vi "_testRTseqBug.vi"(11 "Sequence Context In":refnum<k7>) -> (0 "error out":errorcluster, 3 "Report Text":string)   [LabVIEW 2020]
panel:
  in  "type":enum16{"bool", "number"}(ring)
  in  "stop":bool
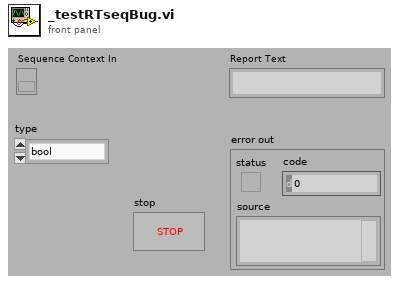
[diagram p1: front panel]
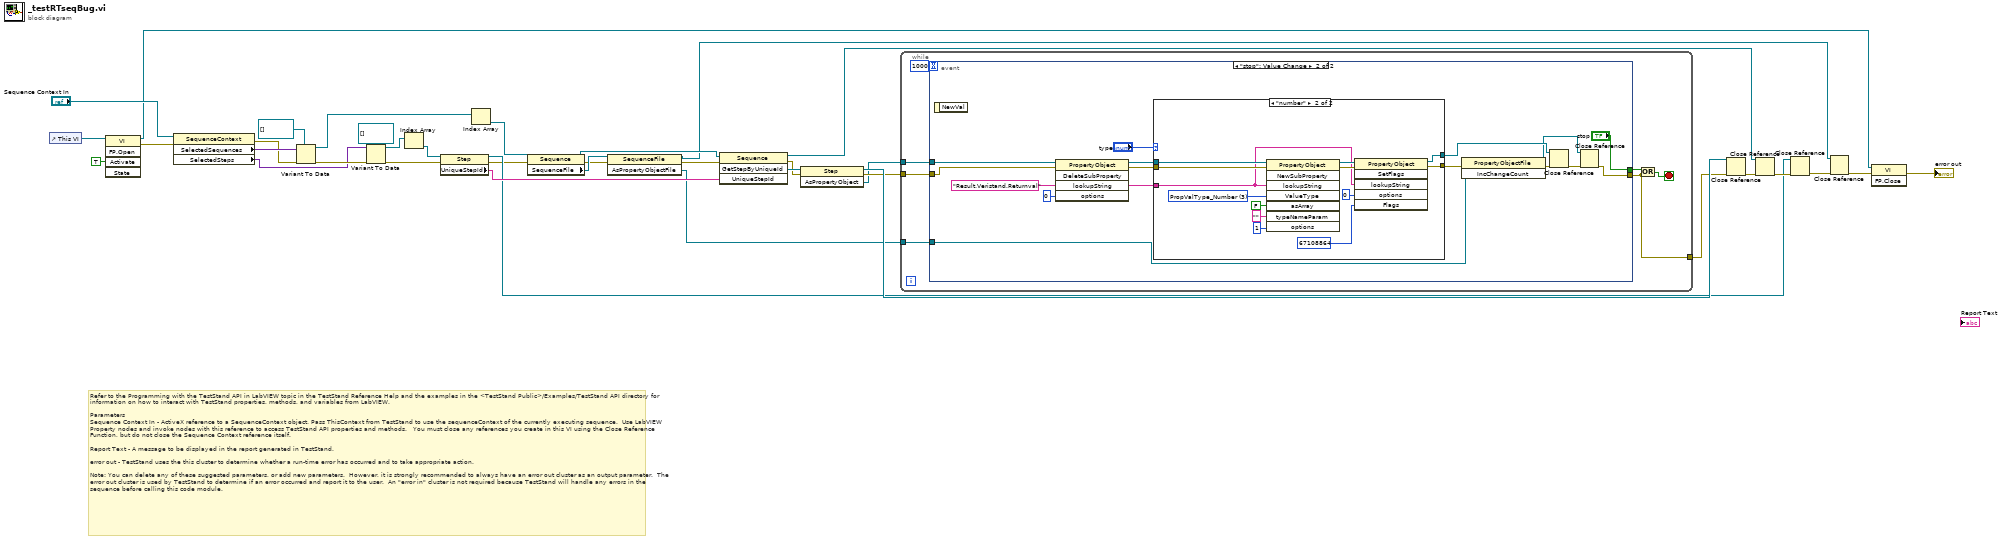
[diagram p0: block diagram]
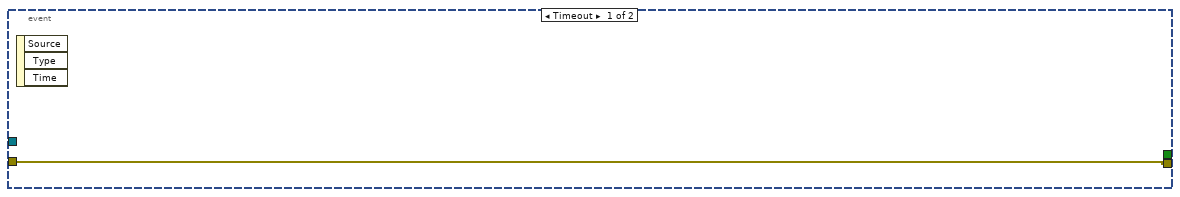
[diagram p2: hidden frame]
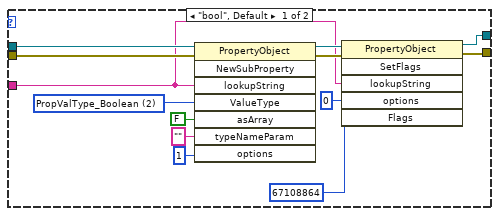
[diagram p3: hidden frame]
diagram:
  # "Refer to the Programming with the TestStand API in LabVIEW topic in the TestStand Reference Help and the examples in the <TestStand Public>/Examples/TestStand API directory for information on how to interact with TestStand properties, methods, and variables from LabVIEW.\n\nParameters\nSequence Context In - ActiveX reference to a SequenceContext object. Pass ThisContext from TestStand to use the sequenceContext of the currently executing sequence.  Use LabVIEW Property nodes and invoke nodes with this reference to access TestStand API properties and methods.   You must close any references you create in this VI using the Close Reference Function, but do not close the Sequence Context reference itself.\n\nReport Text - A message to be displayed in the report generated in TestStand. \n\nerror out - TestStand uses the this cluster to determine whether a run-time error has occurred and to take appropriate action.  \n\nNote: You can delete any of these suggested parameters, or add new parameters.  However, it is strongly recommended to always have an error out cluster as an output parameter.  The error out cluster is used by TestStand to determine if an error occurred and report it to the user.  An \"error in\" cluster is not required because TestStand will handle any errors in the sequence before calling this code module."
  n1 = control-ref of="This VI"() -> (w3:refnum<vi>)
  n2 = invoke class="VI" method="FP.Open"(reference=w3, "Activate"=TRUE ("Activate?")) -> (reference out=w2:refnum<vi>, error out=w4:errorcluster)  [unwired: 3 in, 3 out]
  n3 = property class="SequenceContext"(reference="Sequence Context In", error in=w4) -> (error out=w35:errorcluster, "SelectedSequences"=w36:variant, "SelectedSteps"=w31:variant)  [unwired: 1 out]
  n4 = Variant To Data(error in=w35, type=refnum<k7>[] [] ("Sequence"), Variant=w36) -> (data=w33:refnum<k7>[], error out=w32:errorcluster)
  n5 = Variant To Data(error in=w32, type=refnum<k7>[] [] ("Step"), Variant=w31) -> (data=w29:refnum<k7>[], error out=w27:errorcluster)
  n6 = Index Array(array=w29) -> (element=w28:refnum<k7>)  [unwired: 1 in]
  n7 = property class="Step"(reference=w28, error in=w27) -> (reference out=w19:refnum<k7>, error out=w14:errorcluster, "UniqueStepId"=w26:string)
  n8 = Index Array(array=w33) -> (element=w15:refnum<k7>)  [unwired: 1 in]
  n9 = property class="Sequence"(reference=w15, error in=w14) -> (reference out=w12:refnum<k7>, error out=w11:errorcluster, "SequenceFile"=w13:refnum<k7>)
  n10 = invoke class="SequenceFile" method="AsPropertyObjectFile"(reference=w13, error in=w11) -> (reference out=w8:refnum<k7>, error out=w10:errorcluster, "AsPropertyObjectFile"=w7:refnum<k7>)  [unwired: 1 in]
  n11 = invoke class="Sequence" method="GetStepByUniqueId"(reference=w12, error in=w10, "UniqueStepId"=w26) -> (reference out=w21:refnum<k7>, error out=w24:errorcluster, "GetStepByUniqueId"=w25:refnum<k7>)  [unwired: 1 in, 1 out]
  n12 = invoke class="Step" method="AsPropertyObject"(reference=w25, error in=w24) -> (reference out=w22:refnum<k7>, error out=w18:errorcluster, "AsPropertyObject"=w17:refnum<k7>)  [unwired: 1 in]
  n13 = while {
    tunnel: w18 -> [w44]
    tunnel: w17 -> [w41]
    tunnel: [w39] -> w16
    tunnel: w7 -> [w38]
    stop <- w42 stop-if-true
    n14 = event shown="[1] \"stop\": Value Change" {
      selector: _ -> [_ _]
      dyn-events: _ -> [_ _]
      timeout: 1000 -> [_ _]
      tunnel: w44 -> [w45 w46]
      tunnel: [w45 w52] -> w39
      tunnel: w41 -> [_ w47]
      tunnel: [_ "stop"] -> w40
      tunnel: w38 -> [_ w48]
      event Timeout {
        n15 = event-data() -> ()  [unwired: 1 in, 3 out]
      }
      event "stop": Value Change {
        w57 = "Result.Veristand.Returnval" ("lookupString")
        n16 = event-data() -> ()  [unwired: 1 in, 1 out]
        n17 = invoke class="PropertyObject" method="DeleteSubProperty"(reference=w47, error in=w46, "lookupString"=w57, "options"=0) -> (reference out=w55:refnum<k7>, error out=w59:errorcluster)  [unwired: 1 in, 3 out]
        n18 = case shown="\"number\"" "type" {
          tunnel: w59 -> [w73 w86]
          tunnel: w57 -> [w65 w78]
          tunnel: w55 -> [w70 w83]
          tunnel: [w63 w75] -> w51
          tunnel: [w62 w74] -> w50
          frame "bool", Default {
            w69 = 2 items=["PropValType_Container", "PropValType_String", "PropValType_Boolean", "PropValType_Number", "PropValType_NamedType", "PropValType_Reference", "PropValType_Array", "PropValType_Enum"] ("ValueType")
            n19 = invoke class="PropertyObject" method="NewSubProperty"(reference=w70, error in=w73, "lookupString"=w65, "ValueType"=w69, "asArray"=FALSE, "typeNameParam"="", "options"=1) -> (reference out=w72:refnum<k7>, error out=w71:errorcluster)  [unwired: 1 in, 6 out]
            n20 = invoke class="PropertyObject" method="SetFlags"(reference=w72, error in=w71, "lookupString"=w65, "options"=0, "Flags"=67108864) -> (reference out=w62:refnum<k7>, error out=w63:errorcluster)  [unwired: 1 in, 4 out]
          }
          frame "number" {
            w82 = 3 items=["PropValType_Container", "PropValType_String", "PropValType_Boolean", "PropValType_Number", "PropValType_NamedType", "PropValType_Reference", "PropValType_Array", "PropValType_Enum"] ("ValueType")
            n21 = invoke class="PropertyObject" method="NewSubProperty"(reference=w83, error in=w86, "lookupString"=w78, "ValueType"=w82, "asArray"=FALSE, "typeNameParam"="", "options"=1) -> (reference out=w85:refnum<k7>, error out=w84:errorcluster)  [unwired: 1 in, 6 out]
            n22 = invoke class="PropertyObject" method="SetFlags"(reference=w85, error in=w84, "lookupString"=w78, "options"=0, "Flags"=67108864) -> (reference out=w74:refnum<k7>, error out=w75:errorcluster)  [unwired: 1 in, 4 out]
          }
        }
        n23 = invoke class="PropertyObjectFile" method="IncChangeCount"(reference=w48, error in=w51) -> (reference out=w49:refnum<k7>, error out=w54:errorcluster)  [unwired: 1 in, 1 out]
        n24 = Close Reference(reference=w50, error in (no error)=w54) -> (error out=w53:errorcluster)
        n25 = Close Reference(reference=w49, error in (no error)=w53) -> (error out=w52:errorcluster)
      }
    }
    n26 = Or(x=w40, y=w39) -> (x .or. y?=w42:bool)
  }
  n27 = Close Reference(reference=w22, error in (no error)=w16) -> (error out=w23:errorcluster)
  n28 = Close Reference(reference=w21, error in (no error)=w23) -> (error out=w20:errorcluster)
  n29 = Close Reference(reference=w19, error in (no error)=w20) -> (error out=w9:errorcluster)
  n30 = Close Reference(reference=w8, error in (no error)=w9) -> (error out=w6:errorcluster)
  n31 = invoke class="VI" method="FP.Close"(reference=w2, error in=w6) -> (error out=→"error out":errorcluster)  [unwired: 1 in, 2 out]
